vi "Complex Compact Array to Matrix.vi"(0 "Compact Array":cluster{"Compact Array":cdb[], "array type":i32} {"array type" items=["lower triangular", "upper triangular", "symmetric matrix"]; "Compact Array" format="%.2f"}) -> (1 "Matrix A":T1, 2 "error":i32)   [LabVIEW 2024, in "NI_AALBase.lvlib"]
uses:
  NI_AALBase.lvlib
  ComplexMatrix.ctl
  <resource>/lvanlys.dll
  NI_Matrix.lvlib
panel:
  # "Complex Matrix to Compact Array"
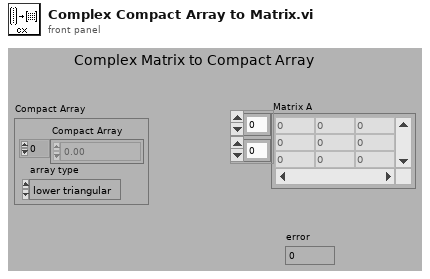
[diagram p1: front panel]
types:
  T1 = typedef "NI_Matrix.lvlib/ComplexMatrix.ctl" = cdb[][]
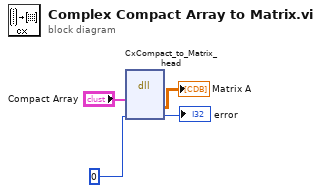
[diagram p0: block diagram]
diagram:
  n1 = dll-call lib="C:/Program Files (x86)/National Instruments/LabVIEW 2024/resource/lvanlys.*" fn="CxCompact_to_Matrix_head"("Compact Array"="Compact Array", 0) -> ("Matrix A"=→"Matrix A":T1, →"error":i32)  [unwired: 6 in, 2 out]
